vi "注释.vi"() -> ()   [LabVIEW 2012]
uses:
  <vilib>/measure/NI_MABase.lvlib
panel:
  in  "sampling info":cluster{"Fs":dbl, "#s":dbl}={"Fs"=1000.0, "#s"=1000.0} caption="采样信息" {"Fs" format="%.2p"}
  in  "停止":bool
  out "波形图":waveform(dbl)(graph)
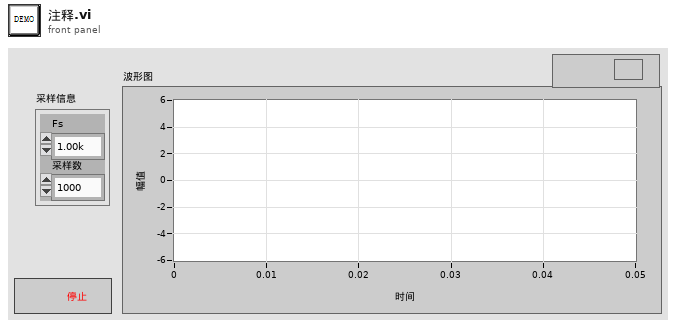
[diagram p1: front panel]
types:
  T1 = typedef "LVAnnotationListTypeDef.ctl" = cluster{"Name":string, "Color":u32, "Style":u8, "Point Style":u8, "Name Visible":bool, "Allow Drag":bool, "Annotation Mode":u32, "Plot":i32, "Index":i32, "Position":cluster{"X":dbl, "Y":dbl}, "X Scale":u32, "Y Scale":u32, "Show Arrow":bool, "Lock Name":bool, "Plot Area":i32, "Label Offset":cluster{"X":dbl, "Y":dbl}}[]
  T2 = cluster{"Name":string, "Color":u32, "Style":u8, "Point Style":u8, "Name Visible":bool, "Allow Drag":bool, "Annotation Mode":u32, "Plot":i32, "Index":i32, "Position":cluster{"X":dbl, "Y":dbl}, "X Scale":u32, "Y Scale":u32, "Show Arrow":bool, "Lock Name":bool, "Plot Area":i32, "Label Offset":cluster{"X":dbl, "Y":dbl}}
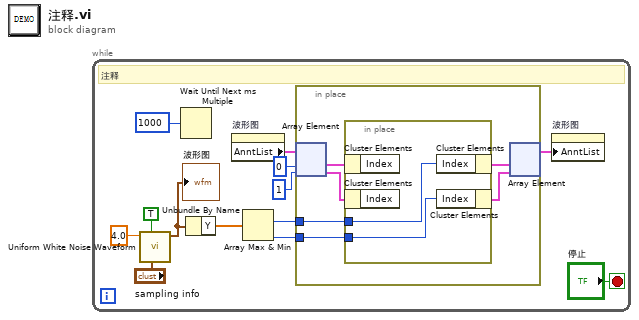
[diagram p0: block diagram]
diagram:
  n1 = while {
    stop <- "停止" stop-if-true
    # "注释"
    n2 = call <vilib>:"Uniform White Noise Waveform.vi"("sampling info"="sampling info", "reset signal"=TRUE, "amplitude"=4.0 ("frequency")) -> ("signal out"=w8:waveform(dbl))  [unwired: 7 in, 1 out]
    "波形图" <- w8
    n3 = Wait Until Next ms Multiple(millisecond multiple=u32 1000 ("毫秒倍数")) -> ()  [unwired: 1 out]
    n4 = Unbundle By Name(w8) -> ("Y"=w7:dbl[])
    n5 = property on="波形图" class="WFGraph (严格)"() -> ("AnntList"=w6:T1)  [unwired: 2 in, 2 out]
    n6 = Array Max & Min(array=w7) -> (max index (indices)=w5:i32, min index (indices)=w4:i32)  [unwired: 2 out]
    n7 = in-place {
      in-place-border: w5 -> [w17]
      in-place-border: w4 -> [w16]
      n8 = in-place-array #1(w6, 0, 1) -> (w19:T2, w18:T2)
      n9 = in-place {
        in-place-border: w17 -> [w21]
        in-place-border: w16 -> [w20]
        n10 = in-place-cluster #2(w19) -> ()  [unwired: 1 out]
        n11 = in-place-cluster #3(w18) -> ()  [unwired: 1 out]
        n12 = in-place-cluster #2("Index"=w21) -> (w15:T2)
        n13 = in-place-cluster #3("Index"=w20) -> (w14:T2)
      }
      n14 = in-place-array #1(w15, w14) -> (w3:T1)  [unwired: 2 out]
    }
    n15 = property on="波形图" class="WFGraph (严格)"("AnntList"=w3) -> ()  [unwired: 2 in, 2 out]
  }
